vi "Igor_SaveWaveToFile.vi"(7 "Path":path, 8 "error in (no error)":errorcluster, 9 "Wave":dbl[](array[numeric]), 10 "Wavename":string) -> (0 "error out":errorcluster, 3 "Path":path)   [LabVIEW 2020]
uses:
  <vilib>/Utility/file.llb/Write To Spreadsheet File (DBL).vi
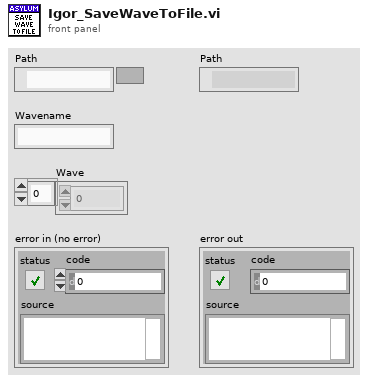
[diagram p1: front panel]
types:
  T1 = enum16{"open", "replace", "create", "open or create", "replace or create", "replace or create with confirmation"}
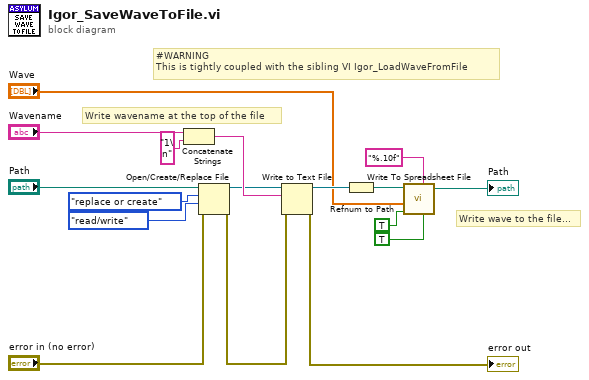
[diagram p0: block diagram]
diagram:
  # "Write wave to the file..."
  # "Write wavename at the top of the file"
  # "#WARNING\nThis is tightly coupled with the sibling VI Igor_LoadWaveFromFile"
  n1 = Concatenate Strings("Wavename", "1\n" ("string")) -> (w11:string)
  n2 = Open/Create/Replace File(file path (use dialog)="Path", error in="error in (no error)", operation (0:open)=T1."replace or create", access (0:read/write)=enum16{"read/write", "read-only", "write-only"}."read/write") -> (refnum out=w10:refnum<file>, error out=w2:errorcluster)  [unwired: 2 in, 1 out]
  n3 = Write to Text File(file (use dialog)=w10, text=w11, error in=w2) -> (refnum out=w12:refnum<file>, error out=→"error out":errorcluster)  [unwired: 1 in, 1 out]
  n4 = Refnum to Path(1:w12) -> (0:w13:path)
  n5 = call-poly <vilib>:"Write To Spreadsheet File.vi"("transpose? (no:F)"=TRUE, "format (%.3f)"="%.10f", "append to file? (new file:F)"=TRUE, "1D data"="Wave", "file path (dialog if empty)"=w13) -> ("new file path (Not A Path if cancelled)"=→"Path":path)  [unwired: 3 in]
